vi "Test.vi"() -> (0 "error out":errorcluster)   [LabVIEW 2022 SP3, in "LoggingActor.lvlib"]
uses:
  LoggingActor.lvlib
  LoggingActor/LoggingActor.lvclass
  <vilib>/ActorFramework/Actor/Actor.lvclass
  <vilib>/ActorFramework/Stop Msg/Stop Msg.lvclass
  C:/Program Files (x86)/National Instruments/LabVIEW 2022/vi.lib/ActorFramework/Actor/Actor.lvclass
  C:/Users/jakub/repos/gh/sw4sys/lv-logging-actor/LoggingActor/Source/LoggingActor/LoggingActor/LoggingActor.lvclass
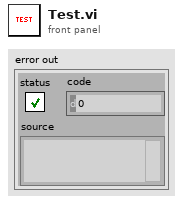
[diagram p1: front panel]
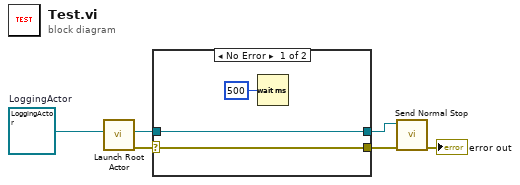
[diagram p0: block diagram]
diagram:
  w5 = refnum<class "LoggingActor.lvclass"> refnum  # LoggingActor
  n1 = call <vilib>:"Launch Root Actor.vi"("Actor"=w5) -> ("error out"=w4:errorcluster, "Actor's Enqueuer"=w3:refnum<class "Message Enqueuer.lvclass">)  [unwired: 9 in]
  n2 = case shown="No Error" w4 {
    selector: w4 -> [w8 w11]
    tunnel: w3 -> [w7 w10]
    tunnel: [w8 w11] -> w2
    tunnel: [w7 w10] -> w1
    frame No Error {
      n3 = Wait (ms)(milliseconds to wait=u32 500) -> ()  [unwired: 1 out]
    }
    frame Error {
    }
  }
  n4 = call <vilib>:"Send Normal Stop.vi"("error in (no error)"=w2, "Message Enqueuer"=w1) -> ("error out"=→"error out":errorcluster)  [unwired: 9 in]
